vi "xiC - IMAQ - Tree_MouseUp.vi"(6 "Coords":T1, 8 "error in (no error)":errorcluster, 11 "Attributes In":T2) -> (0 "error out":errorcluster, 3 "Attributes Out":T2)   [LabVIEW 2013]
uses:
  xiC - IMAQ - Attributes.ctl
  C:/Projects/Cameras3.x/xiLib/xiLIB_64bit/xiLIB/xiCamLib/API/x64/xiApi.NETX64.dll
  xiLIB_64bit/xiLIB/xiCamLib/API/x64/xiApi.NETX64.dll
  xiC - IMAQ - TreeDisplayType.ctl
  <vilib>/Utility/miscctls.llb/LVPoint32TypeDef.ctl
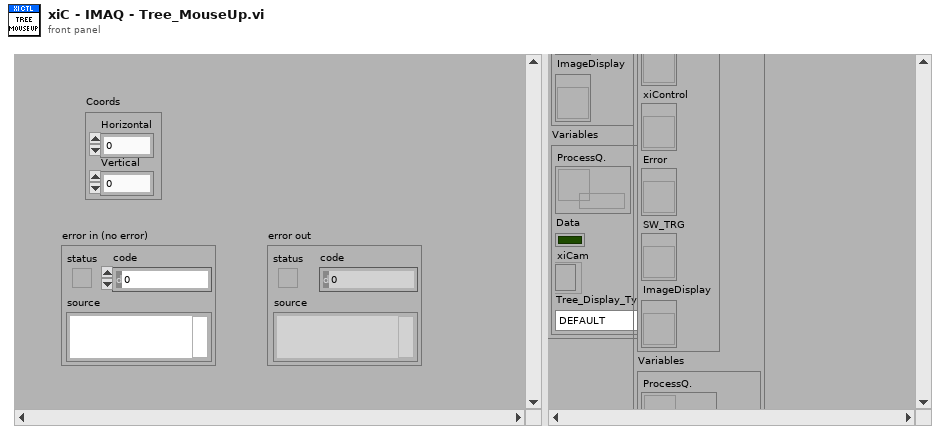
[diagram p1: front panel]
types:
  T1 = typedef "LVPoint32TypeDef.ctl" = cluster{"Horizontal":i32, "Vertical":i32}
  T2 = typedef "xiC - IMAQ - Attributes.ctl" = cluster{"Controls":cluster{"VI Ref.":refnum<vi>, "Tree":refnum<vi>, "Info":refnum<vi>, "PRMName":refnum<vi>, "xiControl":refnum<vi>, "Error":refnum<vi>, "SW_TRG":refnum<vi>, "ImageDisplay":refnum<vi>}, "Variables":cluster{"ProcessQ.":refnum<queue>, "Data":bool, "xiCam":refnum<k24>, "Tree_Display_Type":T3}}
  T3 = typedef "xiC - IMAQ - TreeDisplayType.ctl" = enum16{"DEFAULT", "HIDE_MAX_MIN"}
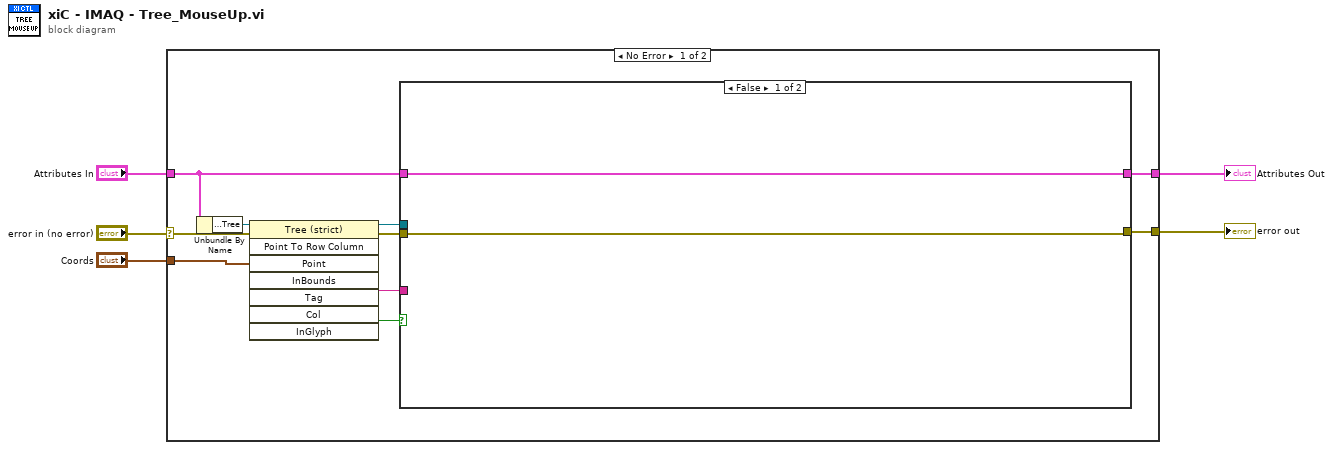
[diagram p0: block diagram]
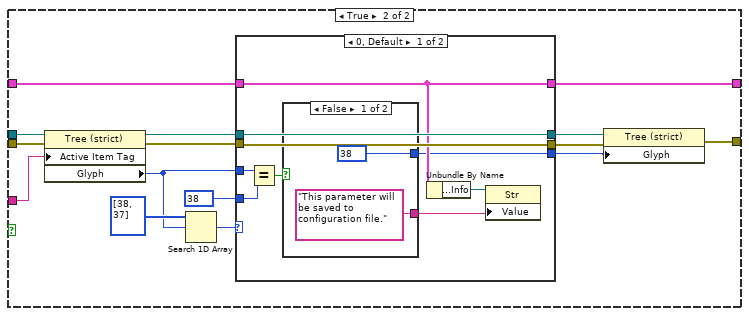
[diagram p2: hidden frame]
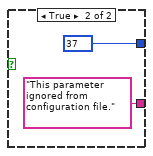
[diagram p3: hidden frame]
diagram:
  n1 = case shown="No Error" "error in (no error)" {
    selector: "error in (no error)" -> [w13 w51]
    tunnel: [w8 w51] -> w4
    tunnel: "Attributes In" -> [w7 w50]
    tunnel: [w6 w50] -> w2
    tunnel: "Coords" -> [w14 _]
    frame No Error {
      n2 = Unbundle By Name(w7) -> ("Controls.Tree"=w15:refnum<vi>)
      n3 = invoke class="Tree (strict)" method="Point To Row Column"(reference=w15, error in=w13, "Point"=w14) -> (reference out=w9:refnum<vi>, error out=w11:errorcluster, "Tag"=w10:string, "InGlyph"=w12:bool)  [unwired: 5 in, 4 out]
      n4 = case shown="False" w12 {
        tunnel: w11 -> [w17 w32]
        tunnel: w10 -> [_ w30]
        tunnel: w9 -> [_ w31]
        tunnel: [w17 w20] -> w8
        tunnel: w7 -> [w16 w19]
        tunnel: [w16 w18] -> w6
        frame False {
        }
        frame True {
          n5 = property class="Tree (strict)"(reference=w31, error in=w32, "Active Item Tag"=w30) -> (reference out=w27:refnum<vi>, error out=w26:errorcluster, "Glyph"=w25:i32)
          n6 = Search 1D Array(1D array=i32[] [38, 37], element=w25) -> (index of element=w28:i32)  [unwired: 1 in]
          n7 = case shown="0, Default" w28 {
            tunnel: w27 -> [w41 w49]
            tunnel: [w41 w49] -> w23
            tunnel: w26 -> [w38 w48]
            tunnel: [w38 w48] -> w22
            tunnel: w25 -> [w40 w47]
            tunnel: 38 -> [w39 _]
            tunnel: [w34 w47] -> w21
            tunnel: w19 -> [w37 w46]
            tunnel: [w37 w46] -> w18
            frame 0, Default {
              n8 = Equal?(x=w40, y=w39) -> (x = y?=w35:bool)
              n9 = case shown="False" w35 {
                tunnel: [38 37] -> w34
                tunnel: ["This parameter will be saved to configuration file." "This parameter ignored from configuration file."] -> w33
                frame False {
                }
                frame True {
                }
              }
              n10 = Unbundle By Name(w37) -> ("Controls.Info"=w36:refnum<vi>)
              n11 = property class="Str"(reference=w36, "Value"=w33) -> ()  [unwired: 1 in, 2 out]
            }
            frame -1 {
            }
          }
          n12 = property class="Tree (strict)"(reference=w23, error in=w22, "Glyph"=w21) -> (error out=w20:errorcluster)  [unwired: 1 out]
        }
      }
    }
    frame Error {
    }
  }
  "error out" <- w4
  "Attributes Out" <- w2
